vi "Manejodedatos.vi"() -> ()   [LabVIEW 2023]
panel:
  out "number":u32
  in  "stop":bool
  out "Array constant":T1
  out "Peso":dbl
  out "Estatura":dbl
  out "Edad":i32
  out "Apellido":string
  out "Nombre":string
  in  "Boolean 3":bool
  in  "Boolean 2":bool
  in  "Boolean":bool
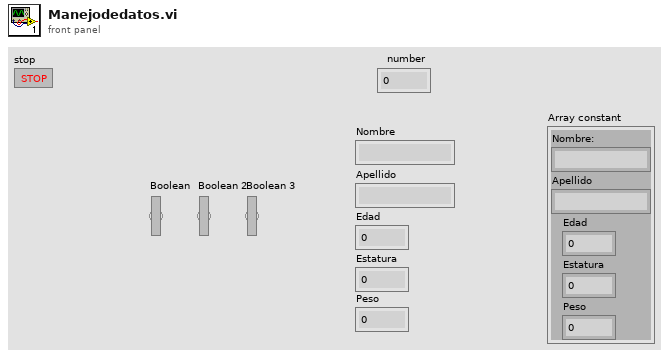
[diagram p1: front panel]
types:
  T1 = cluster{"Nombre:":string, "Apellido":string, "Edad":i32, "Estatura":dbl, "Peso":dbl}
  T2 = cluster{"Nombre:":string, "Apellido":string, "Edad":i32, "Estatura":dbl, "Peso":dbl}[]
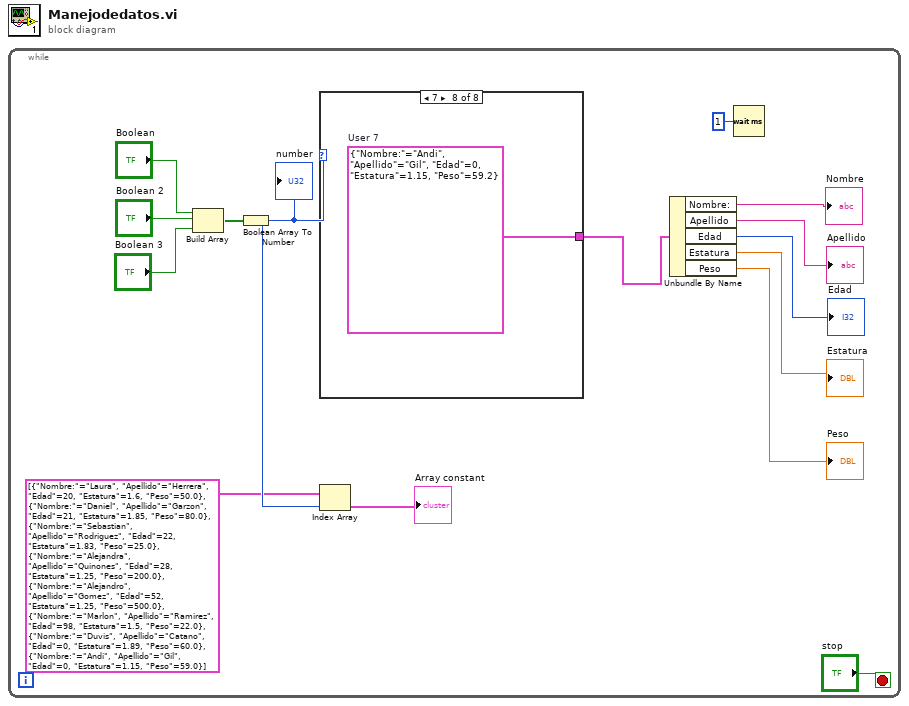
[diagram p0: block diagram]
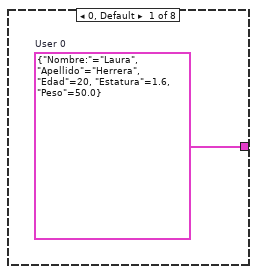
[diagram p2: hidden frame]
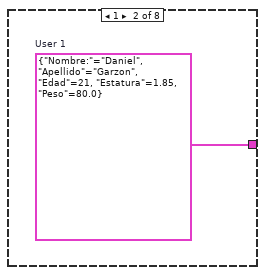
[diagram p3: hidden frame]
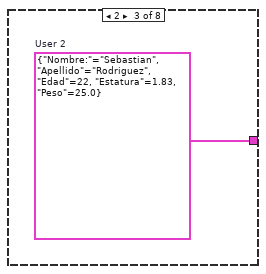
[diagram p4: hidden frame]
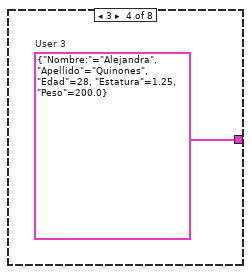
[diagram p5: hidden frame]
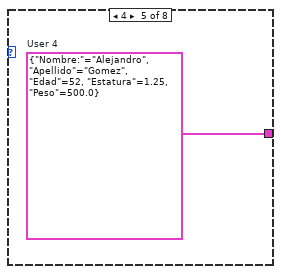
[diagram p6: hidden frame]
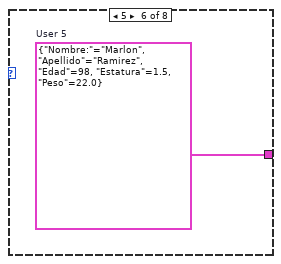
[diagram p7: hidden frame]
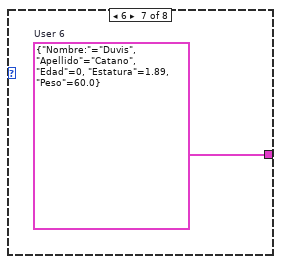
[diagram p8: hidden frame]
diagram:
  n1 = while {
    stop <- "stop" stop-if-true
    n2 = Build Array "Build Array"("Boolean", "Boolean 2", "Boolean 3") -> (w12:bool[])
    n3 = Boolean Array To Number(Boolean array=w12) -> (number=w5:u32)
    "number" <- w5
    n4 = case shown="7" w5 {
      tunnel: [w16 w17 w18 w19 w20 w21 w22 w23] -> w6
      frame 0, Default {
        w16 = T1 {"Nombre:"="Laura", "Apellido"="Herrera", "Edad"=20, "Estatura"=1.6, "Peso"=50.0}  # User 0
      }
      frame 1 {
        w17 = T1 {"Nombre:"="Daniel", "Apellido"="Garzon", "Edad"=21, "Estatura"=1.85, "Peso"=80.0}  # User 1
      }
      frame 2 {
        w18 = T1 {"Nombre:"="Sebastian", "Apellido"="Rodriguez", "Edad"=22, "Estatura"=1.83, "Peso"=25.0}  # User 2
      }
      frame 3 {
        w19 = T1 {"Nombre:"="Alejandra", "Apellido"="Quinones", "Edad"=28, "Estatura"=1.25, "Peso"=200.0}  # User 3
      }
      frame 4 {
        w20 = T1 {"Nombre:"="Alejandro", "Apellido"="Gomez", "Edad"=52, "Estatura"=1.25, "Peso"=500.0}  # User 4
      }
      frame 5 {
        w21 = T1 {"Nombre:"="Marlon", "Apellido"="Ramirez", "Edad"=98, "Estatura"=1.5, "Peso"=22.0}  # User 5
      }
      frame 6 {
        w22 = T1 {"Nombre:"="Duvis", "Apellido"="Catano", "Edad"=0, "Estatura"=1.89, "Peso"=60.0}  # User 6
      }
      frame 7 {
        w23 = T1 {"Nombre:"="Andi", "Apellido"="Gil", "Edad"=0, "Estatura"=1.15, "Peso"=59.2}  # User 7
      }
    }
    n5 = Index Array(array=T2 [{"Nombre:"="Laura", "Apellido"="Herrera", "Edad"=20, "Estatura"=1.6, "Peso"=50.0}, {"Nombre:"="Daniel", "Apellido"="Garzon", "Edad"=21, "Estatura"=1.85, "Peso"=80.0}, {"Nombre:"="Sebastian", "Apellido"="Rodriguez", "Edad"=22, "Estatura"=1.83, "Peso"=25.0}, {"Nombre:"="Alejandra", "Apellido"="Quinones", "Edad"=28, "Estatura"=1.25, "Peso"=200.0}, {"Nombre:"="Alejandro", "Apellido"="Gomez", "Edad"=52, "Estatura"=1.25, "Peso"=500.0}, {"Nombre:"="Marlon", "Apellido"="Ramirez", "Edad"=98, "Estatura"=1.5, "Peso"=22.0}, {"Nombre:"="Duvis", "Apellido"="Catano", "Edad"=0, "Estatura"=1.89, "Peso"=60.0}, {"Nombre:"="Andi", "Apellido"="Gil", "Edad"=0, "Estatura"=1.15, "Peso"=59.0}], index=w5) -> (element=→"Array constant":T1)
    n6 = Unbundle By Name(w6) -> ("Nombre:"=→"Nombre":string, "Apellido"=→"Apellido":string, "Edad"=→"Edad":i32, "Estatura"=→"Estatura":dbl, "Peso"=→"Peso":dbl)
    n7 = Wait (ms)(milliseconds to wait=u32 1) -> ()  [unwired: 1 out]
  }
